vi "Update UI.vi"(8 "error in (no error)":errorcluster, 11 "Main Display in":refnum<class "Main Display.lvclass">) -> (0 "error out":errorcluster, 3 "Main Display out":refnum<class "Main Display.lvclass">)   [LabVIEW 2016, in "Assert API Components.lvlib" / "Assert Display.lvlib" / "Main Display.lvlib" / "Main Display.lvclass"]
uses:
  Main Display.lvclass
  Main Display.lvclass/Main Display.ctl
  Display Configurations/Base Display Configuration.lvclass
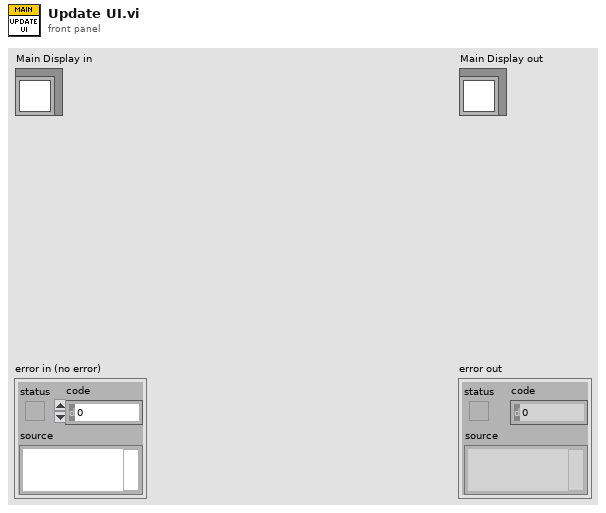
[diagram p1: front panel]
types:
  T1 = typedef "Assert API Components.lvlib/Assert Display.lvlib/Main Display.lvlib/Display Data.ctl" = cluster{"ItemNames":string[][], "Pass Fail Status":bool[], "Display Colours":T2}
  T2 = typedef "Assert API Components.lvlib/Assert Display.lvlib/Main Display.lvlib/Display Colours.ctl" = cluster{"Enable Colours":bool, "Passed Colour":u32, "Failed Colour":u32}
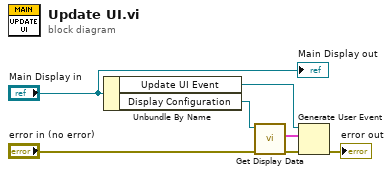
[diagram p0: block diagram]
diagram:
  n1 = Unbundle By Name("Main Display in") -> ("Update UI Event"=w4:refnum<user-event>, "Display Configuration"=w2:refnum<class "Base Display Configuration.lvclass">)
  n2 = call-dynamic "Get Display Data.vi"("error in (no error)"="error in (no error)", "Base Display Configuration in"=w2) -> ("error out"=w3:errorcluster, "Display Data"=w1:T1)  [unwired: 8 in]
  n3 = Generate User Event(user event=w4, event data cluster=w1, error in=w3) -> (error out=→"error out":errorcluster)  [unwired: 1 in, 1 out]
  "Main Display out" <- "Main Display in"
